vi "Initialise Multiple Assert Configuration.vi"(8 "error in (no error)":errorcluster, 11 "GObj Array":refnum<vi>[](array[refnum])) -> (0 "error out":errorcluster, 2 "Modified GObj Array":refnum<vi>[](array[refnum]), 4 "Assert Configuration Array":T1[](array[typedef]), 5 "Valid Assert Count":i32)   [LabVIEW 2016]
uses:
  Assert Build Configuration.ctl
  Core/Assert API Components/Failure Actions.ctl
  <vilib>/Utility/Data Type/Type Definitions/Data Type.ctl
  Core/Assert API Components/Assert API Components.lvlib
  <vilib>/Utility/Data Type/NI_Data Type.lvlib
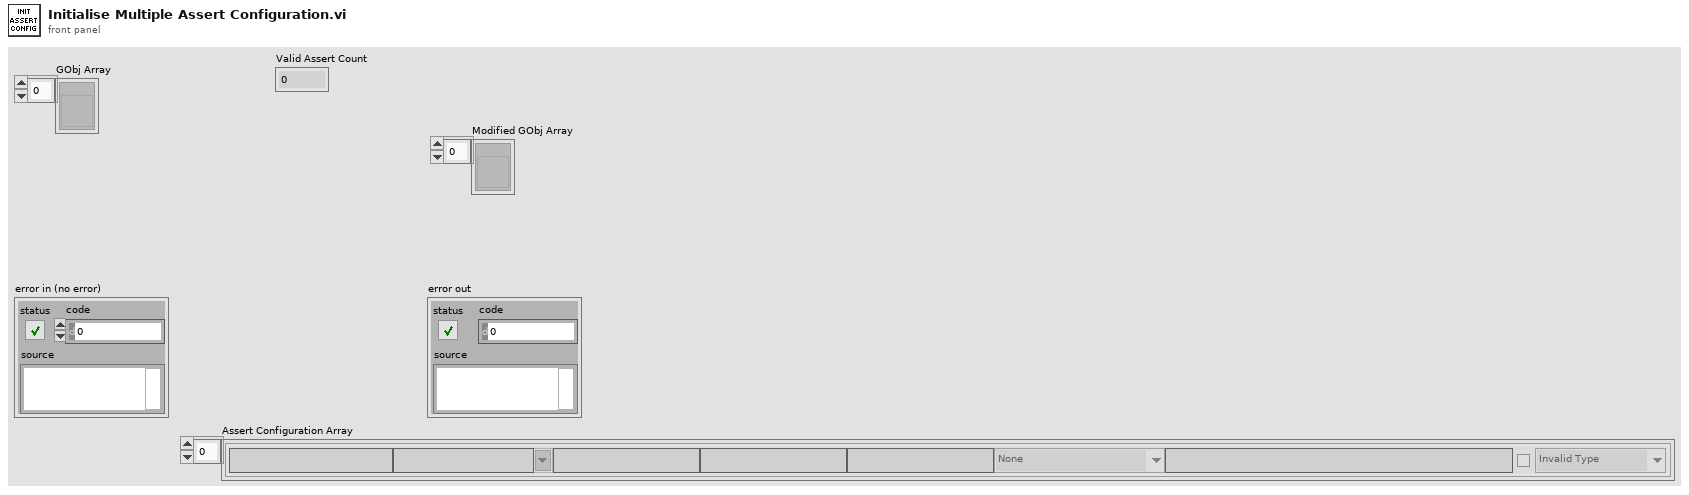
[diagram p1: front panel]
types:
  T1 = typedef "Assert Build Configuration.ctl" = cluster{"Assert Name":string, "Operation":string, "Comparison Value 1":string, "Comparison Value 2":string, "Comment":string, "Default Failure Action":T2, "Description":string, "Operation Display":string, "Active":bool, "Data Type":T3}
  T2 = typedef "Assert API Components.lvlib/Failure Actions.ctl" = enum16{"None", "Log To File", "Pause Execution", "Abort Execution"}
  T3 = typedef "NI_Data Type.lvlib/Data Type.ctl" = enum8{"Invalid Type", "Void", "I8", "I16", "I32", "I64", "U8", "U16", "U32", "U64", "Single Float", "Double Float", "Extended Float", "Single Complex", "Double Complex", "Extended Complex", "Enum U8", "Enum U16", "Enum U32", "Enum U64", "Single Float With Unit", "Double Float With Unit", "Extended Float With Unit", "Single Complex with Unit", "Double Complex with Unit", "Extended Complex with Unit", "Boolean", "String", "Path", "Picture", "Tag", "Array", "Cluster", "Variant", "LV Variant", "Waveform", "Timestamp", "Digital Waveform", "Digital Data", "ExpressData", "Refnum", "External Data", "VI", "Poly VI", "LabVIEW Class Instance", "Fixed Point"}
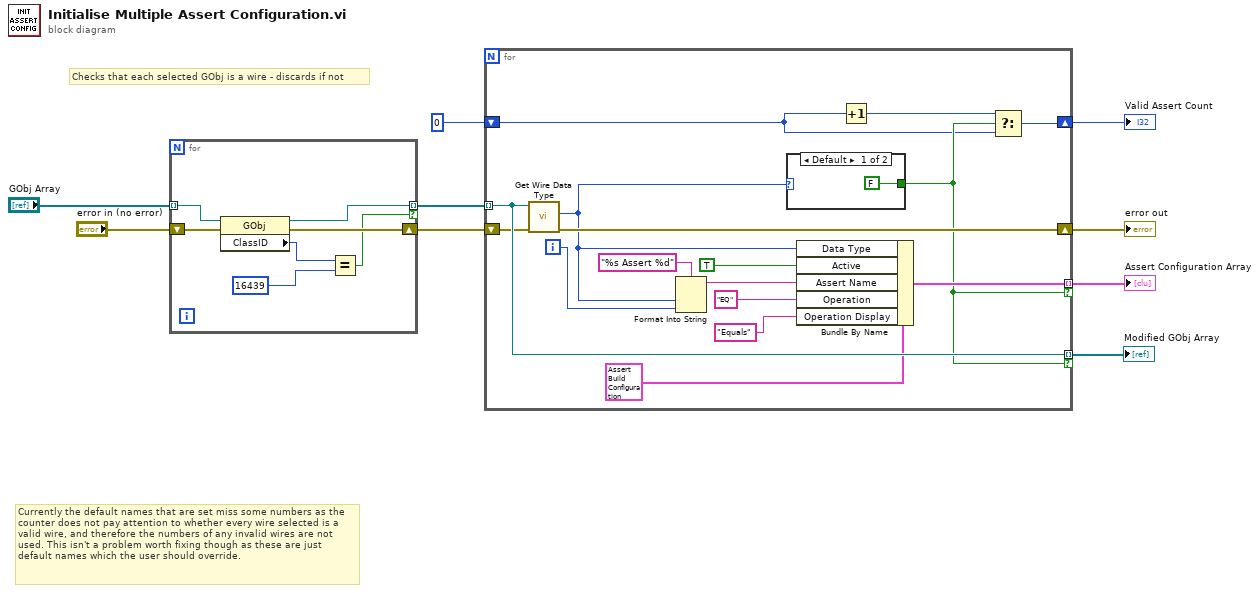
[diagram p0: block diagram]
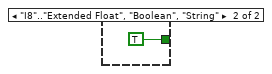
[diagram p2: hidden frame]
diagram:
  # "Checks that each selected GObj is a wire - discards if not"
  # "Currently the default names that are set miss some numbers as the counter does not pay attention to whether every wire selected is a valid wire, and therefore the numbers of any invalid wires are not used. This isn't a problem worth fixing though as these are just default names which the user should override."
  n1 = for {
    tunnel: [w14] -> w2 mode=indexing if=w10
    tunnel: "GObj Array" -> [w13] mode=indexing
    shift-right: [w15] -> w3
    shift-left: "error in (no error)" -> [w16]
    n2 = property class="GObj"(reference=w13, error in=w16) -> (reference out=w14:refnum<vi>, error out=w15:errorcluster, "ClassID"=w12:u32)
    n3 = Equal?(x=w12, y=u32 16439) -> (x = y?=w10:bool)
  }
  n4 = for {
    tunnel: [w32] -> w5 mode=indexing if=w21
    tunnel: w2 -> [w30] mode=indexing
    tunnel: [w30] -> w6 mode=indexing if=w21
    shift-right: [w26] -> w8
    shift-left: w3 -> [w27]
    shift-right: [w18] -> w7
    shift-left: 0 -> [w19]
    i -> [w28]
    n5 = call "Get Wire Data Type.vi"("error in (no error)"=w27, "Wire ref in"=w30) -> ("error out"=w26:errorcluster, "Type"=w17:T3)  [unwired: 7 in, 1 out]
    n6 = Format Into String(format string="%s Assert %d", w17, w28) -> (resulting string=w31:string)  [unwired: 2 in, 1 out]
    n7 = case shown="Default" w17 {
      tunnel: [FALSE TRUE] -> w21
      frame Default {
      }
      frame "I8".."Extended Float", "Boolean", "String" {
      }
    }
    n8 = Bundle By Name(cluster=T1 {"Assert Name"="", "Operation"="", "Comparison Value 1"="", "Comparison Value 2"="", "Comment"="", "Default Failure Action"=enum."None", "Description"="", "Operation Display"="", "Active"=FALSE, "Data Type"=enum."Invalid Type"} ("Assert Build Configuration"), "Data Type"=w17, "Active"=TRUE, "Assert Name"=w31, "Operation"="EQ", "Operation Display"="Equals") -> (w32:T1)
    n9 = Increment(x=w19) -> (x+1=w20:i32)
    n10 = Select(t=w20, s=w21, f=w19) -> (s? t:f=w18:i32)
  }
  "error out" <- w8
  "Valid Assert Count" <- w7
  "Modified GObj Array" <- w6
  "Assert Configuration Array" <- w5
